vi "readVoltFile.vi"(2 "error in (no error)":errorcluster, 3 "Path":path) -> (0 "error out":errorcluster, 1 "Array":sgl[](array[numeric]))   [LabVIEW 2016]
uses:
  <vilib>/Utility/file.llb/Read Delimited Spreadsheet (DBL).vi
  <vilib>/Analysis/Matrix/Numeric/Conversions/Matrix To Array - RM.vi
  <vilib>/Analysis/Matrix/NI_Matrix.lvlib
panel:
  out "product":i32
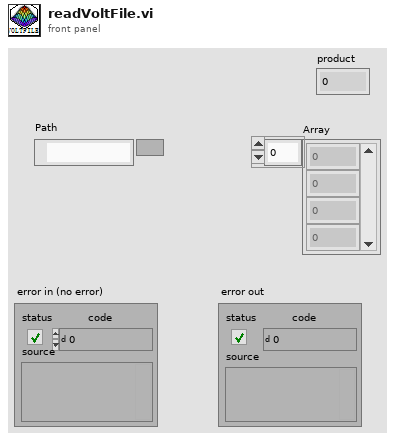
[diagram p1: front panel]
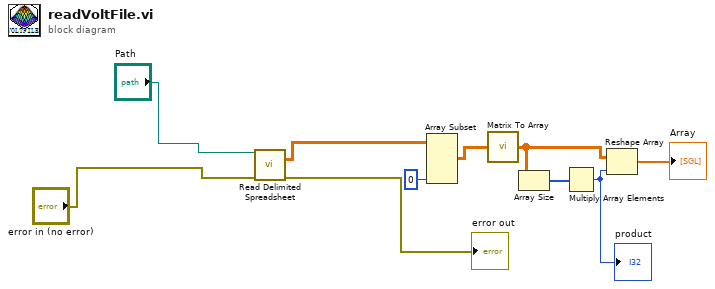
[diagram p0: block diagram]
diagram:
  n1 = call-poly <vilib>:"Read Delimited Spreadsheet.vi"("file path (dialog if empty)"="Path", "error in (no error)"="error in (no error)") -> ("all rows"=w1:dbl[][], "error out"=→"error out":errorcluster)  [unwired: 8 in, 4 out]
  n2 = Array Subset(array=w1, length (col)=0 ("column N")) -> (w7:dbl[][])  [unwired: 3 in]
  n3 = call-poly <vilib>:"Matrix To Array.vi"("Real Matrix"=w7) -> ("Real 2D Array"=w4:dbl[][])
  n4 = Array Size(array=w4) -> (size(s)=w6:i32[])
  n5 = Multiply Array Elements(1:w6) -> (0:w5:i32)
  "product" <- w5
  n6 = Reshape Array(w4, w5) -> (→"Array":dbl[])
